vi "Error to log options.vi"(11 "error in (no error)":errorcluster) -> (2 "Logging level":T1=enum."INFO", 3 "Options":T2={"timestamp (now)"=0.0, "Call chain (here)"="", "Count (1)"=1, "Font (override)"={"Font Name"="", "Size"=0, "Bold"=FALSE, "Italic"=FALSE, "Underline"=FALSE, "Strikeout"=FALSE, "Color"=0}, "Add row separator? (T)"=TRUE})   [LabVIEW 2020, in "Blue Easy HTTP OpenSource.lvlib"]
uses:
  Blue Easy HTTP OpenSource.lvlib
  <userlib>/Blue Origin/BlueLogParent_OpenSource/BlueLogParentClass/BlueLogParentOptions.ctl
  <userlib>/Blue Origin/BlueLogParent_OpenSource/BlueLogParentClass/BlueLogParentFont.ctl
  <userlib>/Blue Origin/BlueLogParent_OpenSource/BlueLogParentClass/BlueLogParentLevel.ctl
  <userlib>/Blue Origin/BlueLogParent_OpenSource/BlueLogParentClass/BlueLogParent_OpenSource.lvclass
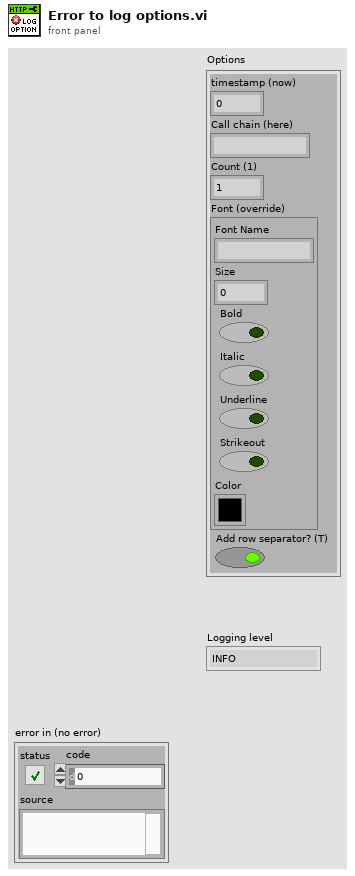
[diagram p1: front panel]
types:
  T1 = typedef "BlueLogParent_OpenSource.lvclass/BlueLogParentLevel.ctl" = enum16{"DEBUG", "INFO", "WARNING", "ERROR", "CRITICAL"}
  T2 = typedef "BlueLogParent_OpenSource.lvclass/BlueLogParentOptions.ctl" = cluster{"timestamp (now)":dbl, "Call chain (here)":string, "Count (1)":u16, "Font (override)":T3, "Add row separator? (T)":bool}
  T3 = typedef "BlueLogParent_OpenSource.lvclass/BlueLogParentFont.ctl" = cluster{"Font Name":string, "Size":u16, "Bold":bool, "Italic":bool, "Underline":bool, "Strikeout":bool, "Color":u32}
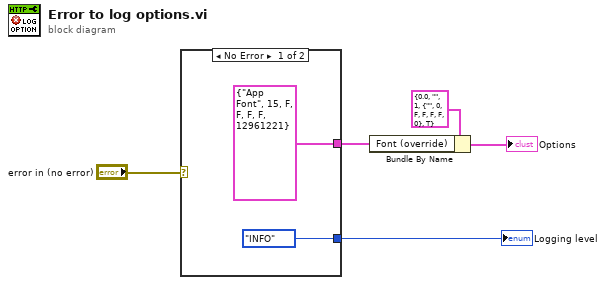
[diagram p0: block diagram]
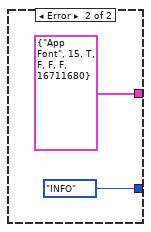
[diagram p2: hidden frame]
diagram:
  n1 = case shown="No Error" "error in (no error)" {
    tunnel: [T3 {"Font Name"="App Font", "Size"=15, "Bold"=FALSE, "Italic"=FALSE, "Underline"=FALSE, "Strikeout"=FALSE, "Color"=12961221} ("Font (override)") T3 {"Font Name"="App Font", "Size"=15, "Bold"=TRUE, "Italic"=FALSE, "Underline"=FALSE, "Strikeout"=FALSE, "Color"=16711680} ("Font (override)")] -> w3
    tunnel: [BlueLogParentLevel."INFO" ("Logging level") BlueLogParentLevel."INFO" ("Logging level")] -> w1
    frame No Error {
    }
    frame Error {
    }
  }
  "Logging level" <- w1
  n2 = Bundle By Name(cluster=T2 {"timestamp (now)"=0.0, "Call chain (here)"="", "Count (1)"=1, "Font (override)"={"Font Name"="", "Size"=0, "Bold"=FALSE, "Italic"=FALSE, "Underline"=FALSE, "Strikeout"=FALSE, "Color"=0}, "Add row separator? (T)"=TRUE} ("Options"), "Font (override)"=w3) -> (→"Options":T2)
